vi "fgv_sva_mode.vi"(8 "Error in":errorcluster, 9 "cal_file_in":string, 10 "data_in":T1, 11 "mode":string(combo)="Get") -> (0 "error out":errorcluster, 1 "cal_file_out":string, 2 "data_out":T1)   [LabVIEW 2025]
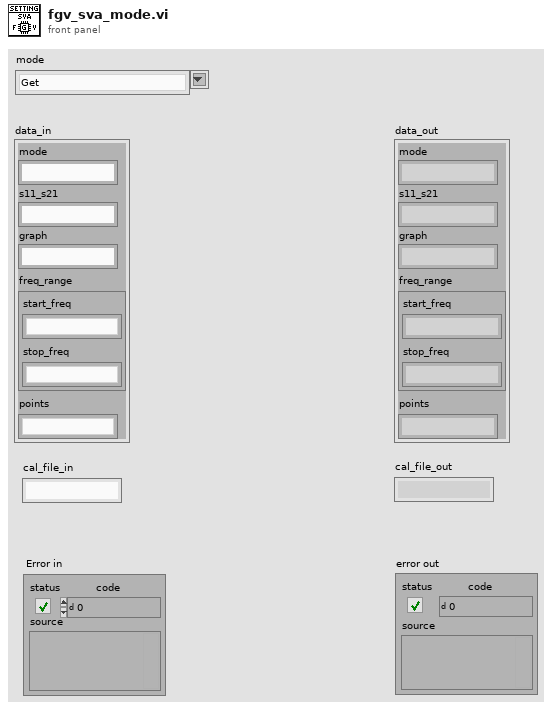
[diagram p1: front panel]
types:
  T1 = cluster{"mode":string, "s11_s21":string, "graph":string, "freq_range":cluster{"start_freq":string, "stop_freq":string}, "points":string}
  T2 = cluster{"mode":string, "s11_s21":string, "graph":string, cluster{"start_freq":string, "stop_freq":string}, "points":string}
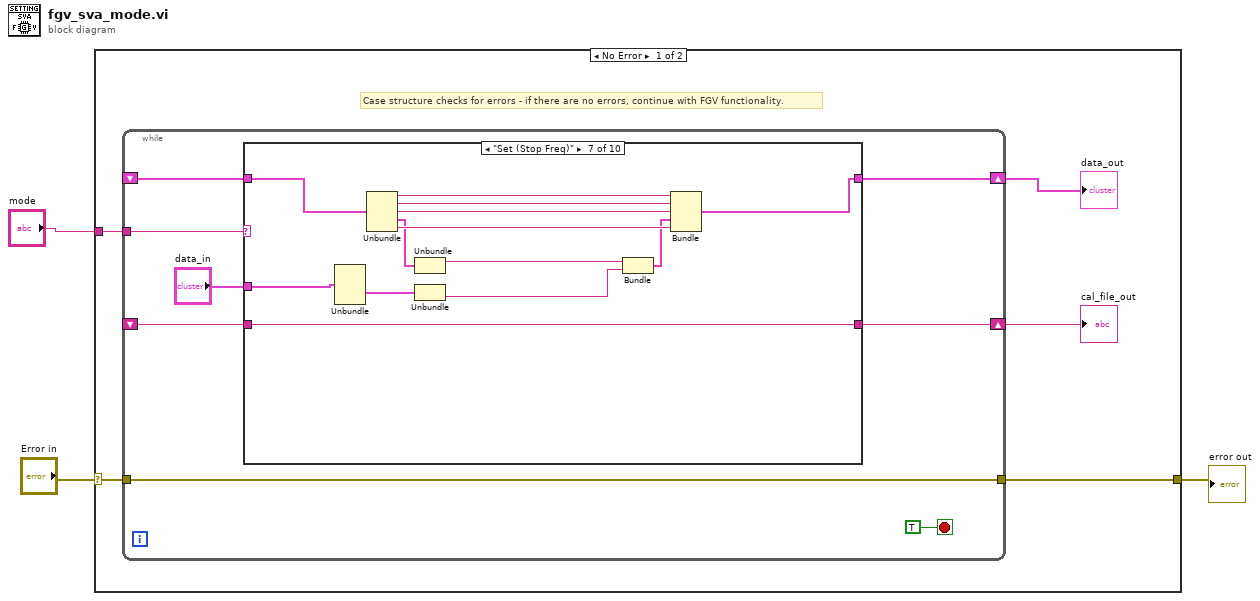
[diagram p0: block diagram]
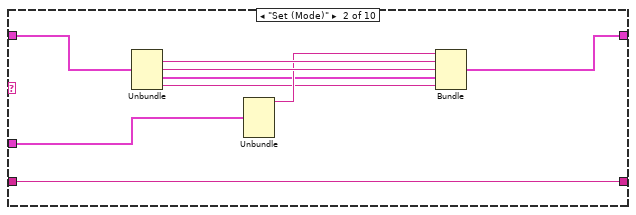
[diagram p3: hidden frame]
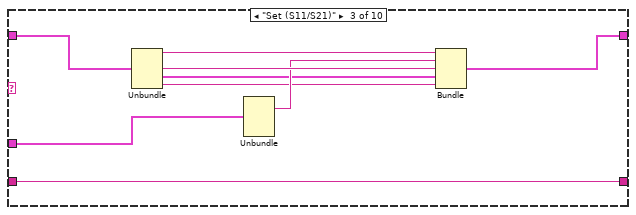
[diagram p4: hidden frame]
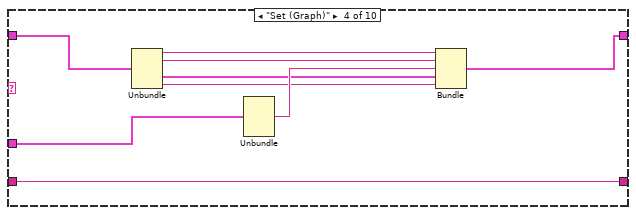
[diagram p5: hidden frame]
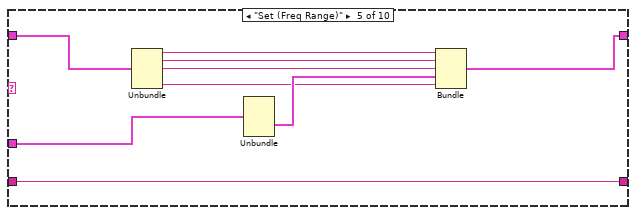
[diagram p6: hidden frame]
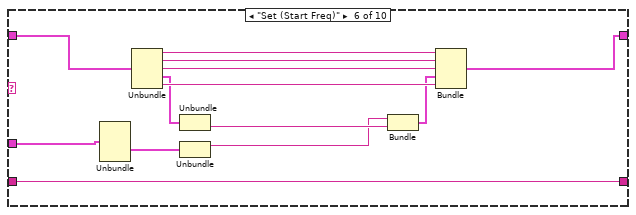
[diagram p7: hidden frame]
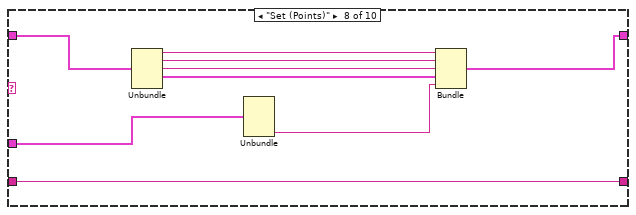
[diagram p8: hidden frame]
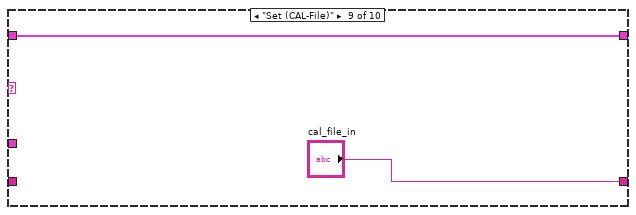
[diagram p9: hidden frame]
diagram:
  n1 = case shown="No Error" "Error in" {
    selector: "Error in" -> [w8 w94]
    tunnel: [w7 w94] -> w2
    tunnel: "mode" -> [w6 _]
    frame No Error {
      # "Case structure checks for errors - if there are no errors, continue with FGV functionality."
      n2 = while {
        tunnel: w8 -> [w15]
        tunnel: [w15] -> w7
        tunnel: w6 -> [w14]
        shift-right: [w13] -> w4
        shift-left: _ -> [w12]
        shift-right: [w11] -> w5
        shift-left: _ -> [w10]
        stop <- TRUE stop-if-true
        n3 = case shown="\"Set (Stop Freq)\"" w14 {
          tunnel: [w18 w22 w34 w44 w53 w66 w79 w88 w90 w93] -> w13
          tunnel: w12 -> [w18 w27 w33 w42 w51 w64 w77 w86 w90 _]
          tunnel: "data_in" -> [_ w23 w35 w43 w52 w65 w78 w87 _ w93]
          tunnel: [w17 w21 w30 w39 w49 w62 w75 w84 "cal_file_in" w92] -> w11
          tunnel: w10 -> [w17 w21 w30 w39 w49 w62 w75 w84 _ w92]
          frame "Get", Default {
          }
          frame "Set (Mode)" {
            n4 = Unbundle(w27) -> ("s11_s21"=w26:string, "graph"=w25:string, "freq_range"=w20:cluster{"start_freq":string, "stop_freq":string}, "points"=w19:string)  [unwired: 1 out]
            n5 = Unbundle(w23) -> ("mode"=w24:string)  [unwired: 4 out]
            n6 = Bundle("mode"=w24, "s11_s21"=w26, "graph"=w25, "freq_range"=w20, "points"=w19) -> (w22:T1)  [unwired: 1 in]
          }
          frame "Set (S11/S21)" {
            n7 = Unbundle(w33) -> ("mode"=w32:string, "graph"=w36:string, "freq_range"=w29:cluster{"start_freq":string, "stop_freq":string}, "points"=w28:string)  [unwired: 1 out]
            n8 = Unbundle(w35) -> ("s11_s21"=w31:string)  [unwired: 4 out]
            n9 = Bundle("mode"=w32, "s11_s21"=w31, "graph"=w36, "freq_range"=w29, "points"=w28) -> (w34:T1)  [unwired: 1 in]
          }
          frame "Set (Graph)" {
            n10 = Unbundle(w42) -> ("mode"=w41:string, "s11_s21"=w45:string, "freq_range"=w38:cluster{"start_freq":string, "stop_freq":string}, "points"=w37:string)  [unwired: 1 out]
            n11 = Unbundle(w43) -> ("graph"=w40:string)  [unwired: 4 out]
            n12 = Bundle("mode"=w41, "s11_s21"=w45, "graph"=w40, "freq_range"=w38, "points"=w37) -> (w44:T1)  [unwired: 1 in]
          }
          frame "Set (Freq Range)" {
            n13 = Unbundle(w51) -> ("mode"=w50:string, "s11_s21"=w54:string, "graph"=w48:string, "points"=w46:string)  [unwired: 1 out]
            n14 = Unbundle(w52) -> ("freq_range"=w47:cluster{"start_freq":string, "stop_freq":string})  [unwired: 4 out]
            n15 = Bundle("mode"=w50, "s11_s21"=w54, "graph"=w48, "freq_range"=w47, "points"=w46) -> (w53:T1)  [unwired: 1 in]
          }
          frame "Set (Start Freq)" {
            n16 = Unbundle(w65) -> ("freq_range"=w56:cluster{"start_freq":string, "stop_freq":string})  [unwired: 4 out]
            n17 = Unbundle(w64) -> ("mode"=w63:string, "s11_s21"=w67:string, "graph"=w61:string, "freq_range"=w59:cluster{"start_freq":string, "stop_freq":string}, "points"=w60:string)
            n18 = Unbundle(w59) -> ("stop_freq"=w57:string)  [unwired: 1 out]
            n19 = Unbundle(w56) -> ("start_freq"=w55:string)  [unwired: 1 out]
            n20 = Bundle("start_freq"=w55, "stop_freq"=w57) -> (w58:cluster{"start_freq":string, "stop_freq":string})  [unwired: 1 in]
            n21 = Bundle("mode"=w63, "s11_s21"=w67, "graph"=w61, w58, "points"=w60) -> (w66:T2)  [unwired: 1 in]
          }
          frame "Set (Stop Freq)" {
            n22 = Unbundle(w78) -> ("freq_range"=w70:cluster{"start_freq":string, "stop_freq":string})  [unwired: 4 out]
            n23 = Unbundle(w77) -> ("mode"=w76:string, "s11_s21"=w80:string, "graph"=w74:string, "freq_range"=w72:cluster{"start_freq":string, "stop_freq":string}, "points"=w73:string)
            n24 = Unbundle(w72) -> ("start_freq"=w69:string)  [unwired: 1 out]
            n25 = Unbundle(w70) -> ("stop_freq"=w68:string)  [unwired: 1 out]
            n26 = Bundle("start_freq"=w69, "stop_freq"=w68) -> (w71:cluster{"start_freq":string, "stop_freq":string})  [unwired: 1 in]
            n27 = Bundle("mode"=w76, "s11_s21"=w80, "graph"=w74, w71, "points"=w73) -> (w79:T2)  [unwired: 1 in]
          }
          frame "Set (Points)" {
            n28 = Unbundle(w86) -> ("mode"=w85:string, "s11_s21"=w89:string, "graph"=w83:string, "freq_range"=w81:cluster{"start_freq":string, "stop_freq":string})  [unwired: 1 out]
            n29 = Unbundle(w87) -> ("points"=w82:string)  [unwired: 4 out]
            n30 = Bundle("mode"=w85, "s11_s21"=w89, "graph"=w83, "freq_range"=w81, "points"=w82) -> (w88:T1)  [unwired: 1 in]
          }
          frame "Set (CAL-File)" {
          }
          frame "Set All" {
          }
        }
      }
      "cal_file_out" <- w5
      "data_out" <- w4
    }
    frame Error {
      # "Case structure checks for errors - if there's an errorr, do nothing except pass the error back out"
    }
  }
  "error out" <- w2
